vi "Update from Process.vi"(8 "error in (no error)":errorcluster, 10 "Value":dbl, 11 "Running in":refnum<class "Running.lvclass">) -> (0 "error out":errorcluster, 3 "Process State out":refnum<class "State Actor.lvclass">)   [LabVIEW 2013, in "Process States.lvlib" / "Running.lvclass"]
doc: "This override maintains a count and running average of all values received from Process Actor. It also sends a Log Event message to the UI containing the value and its index in the stream. When the third value is received, this method invokes the Go to Idle method."
uses:
  Running.lvclass
  State Actor/State Actor.lvclass
  <vilib>/ActorFramework/Actor/Actor.lvclass/Actor.ctl
  Running.lvclass/Running.ctl
  State Pattern UI/Log Event Msg/Log Event Msg.lvclass/Log Event Msg.ctl
  <vilib>/ActorFramework/Message Enqueuer/Message Enqueuer.lvclass/Message Enqueuer.ctl
  <vilib>/ActorFramework/Message Enqueuer/Enqueue.vi
  <vilib>/ActorFramework/Message Priority Queue/Priority Enqueue.vi
  State Pattern UI/Log Event Msg/Log Event Msg.lvclass
  <vilib>/ActorFramework/Actor/Actor.lvclass
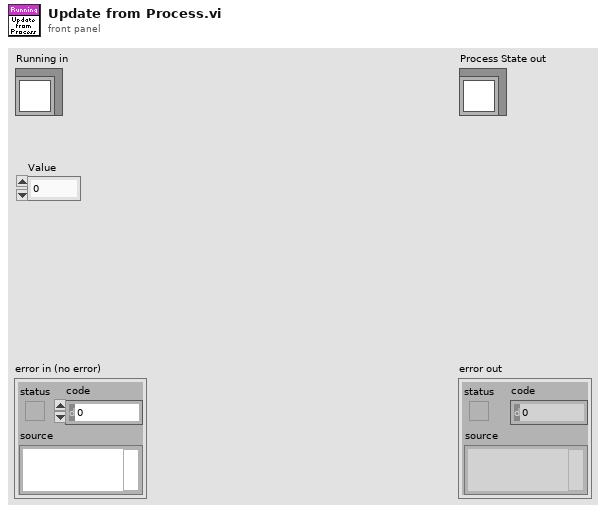
[diagram p1: front panel]
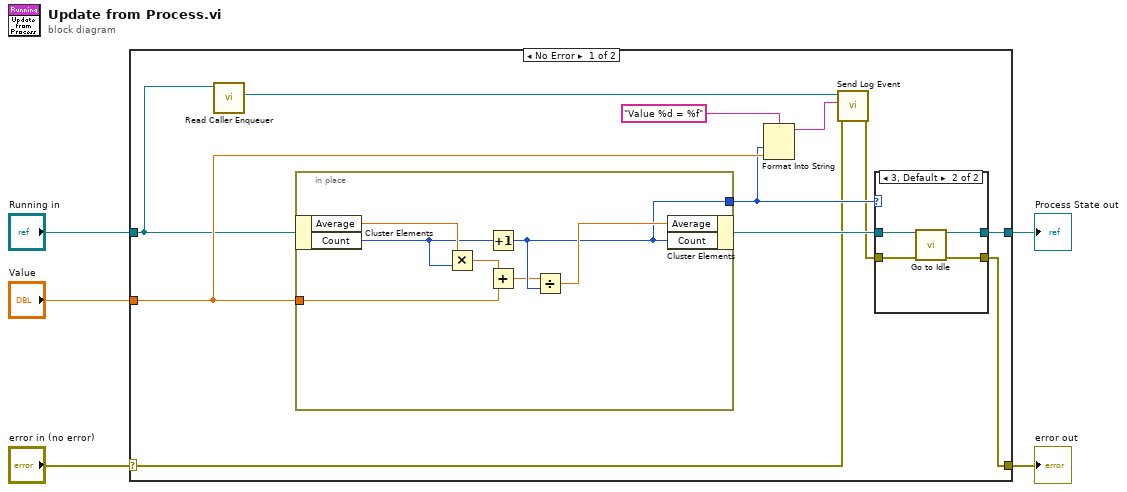
[diagram p0: block diagram]
diagram:
  n1 = case shown="No Error" "error in (no error)" {
    selector: "error in (no error)" -> [w8 w31]
    tunnel: [w6 w31] -> w4
    tunnel: [w15 w30] -> w2
    tunnel: "Running in" -> [w9 w30]
    tunnel: "Value" -> [w13 _]
    frame No Error {
      n2 = call <vilib>:"Read Caller Enqueuer.vi"("Actor"=w9) -> ("Caller Enqueuer"=w10:refnum<class "Message Enqueuer.lvclass">)  [unwired: 10 in]
      n3 = in-place {
        in-place-border: w13 -> [w27]
        in-place-border: [w25] -> w12
        n4 = in-place-cluster #1(w9) -> ("Average"=w29:dbl, "Count"=w28:i32)
        n5 = Multiply(x=w29, y=w28) -> (x*y=w24:dbl)
        n6 = Increment(x=w28) -> (x+1=w25:i32)
        n7 = Add(x=w24, y=w27) -> (x+y=w23:dbl)
        n8 = Divide(x=w23, y=w25) -> (x/y=w26:dbl)
        n9 = in-place-cluster #1("Average"=w26, "Count"=w25) -> (w16:refnum<class "Running.lvclass">)
      }
      n10 = Format Into String(format string="Value %d = %f", w12, w13) -> (resulting string=w11:string)  [unwired: 2 in, 1 out]
      n11 = call "Send Log Event.vi"("error in (no error)"=w8, "Event Text"=w11, "Message Enqueuer"=w10) -> ("error out"=w7:errorcluster)  [unwired: 8 in]
      n12 = case shown="3, Default" w12 {
        tunnel: w16 -> [w18 w22]
        tunnel: [w18 w21] -> w15
        tunnel: w7 -> [w17 w20]
        tunnel: [w17 w19] -> w6
        frame 1, 2 {
        }
        frame 3, Default {
          n13 = call-dynamic "Go to Idle.vi"("error in (no error)"=w20, "Process State in"=w22) -> ("error out"=w19:errorcluster, "Process State out"=w21:refnum<class "State Actor.lvclass">)  [unwired: 8 in]
        }
      }
    }
    frame Error {
    }
  }
  "error out" <- w4
  "Process State out" <- w2
